vi "Read RutaImagenes.vi"(8 "error in (no error)":errorcluster, 11 "Simulada in":refnum<class "Simulada.lvclass">) -> (0 "error out":errorcluster, 2 "RutaImagenes":path, 3 "Simulada out":refnum<class "Simulada.lvclass">)   [LabVIEW 2020, in "Simulada.lvclass"]
uses:
  Simulada.lvclass
  Simulada.lvclass/Simulada.ctl
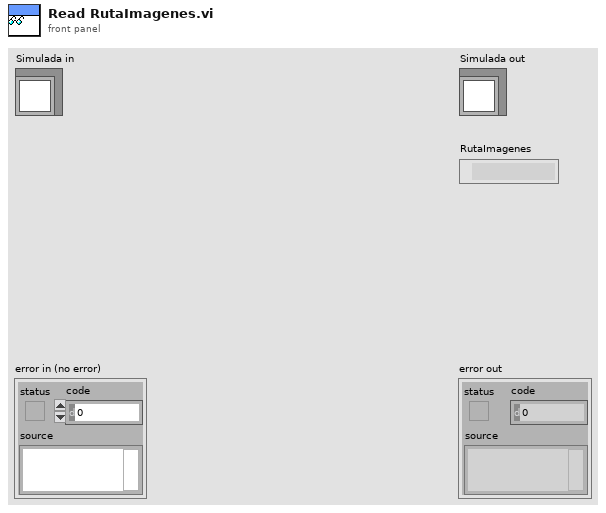
[diagram p1: front panel]
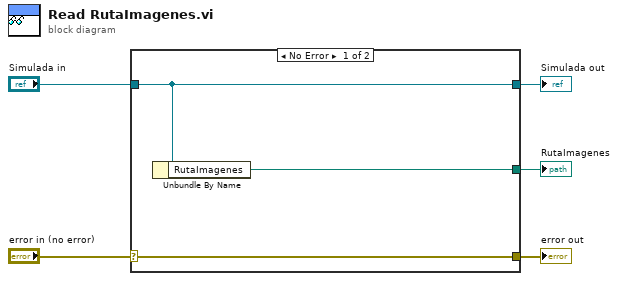
[diagram p0: block diagram]
diagram:
  n1 = case shown="No Error" "error in (no error)" {
    selector: "error in (no error)" -> [w8 w9]
    tunnel: [w8 w9] -> w4
    tunnel: [w7 w10] -> w2
    tunnel: "Simulada in" -> [w7 w10]
    tunnel: [w6 _] -> w1
    frame No Error {
      n2 = Unbundle By Name(w7) -> ("RutaImagenes"=w6:path)
    }
    frame Error {
    }
  }
  "error out" <- w4
  "Simulada out" <- w2
  "RutaImagenes" <- w1
